vi "GetEdgeMenu.vi"(0 "reference":refnum<class "AbstractEdge.lvclass">, 5 "error in (no error)":errorcluster) -> (14 "reference out":refnum<class "AbstractEdge.lvclass">, 15 "MenuOptions":string[](array[string]), 19 "error out":errorcluster)   [LabVIEW 2014, in "AbstractEdge.lvclass"]
doc: "GetEdgeMenu"
uses:
  <resource>/Framework/Providers/Open_GDS/UML/AbstractEdge_class/AbstractEdge.lvclass
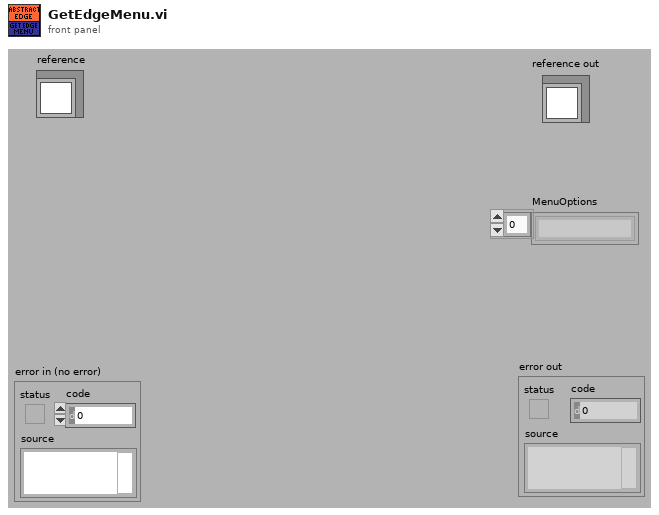
[diagram p1: front panel]
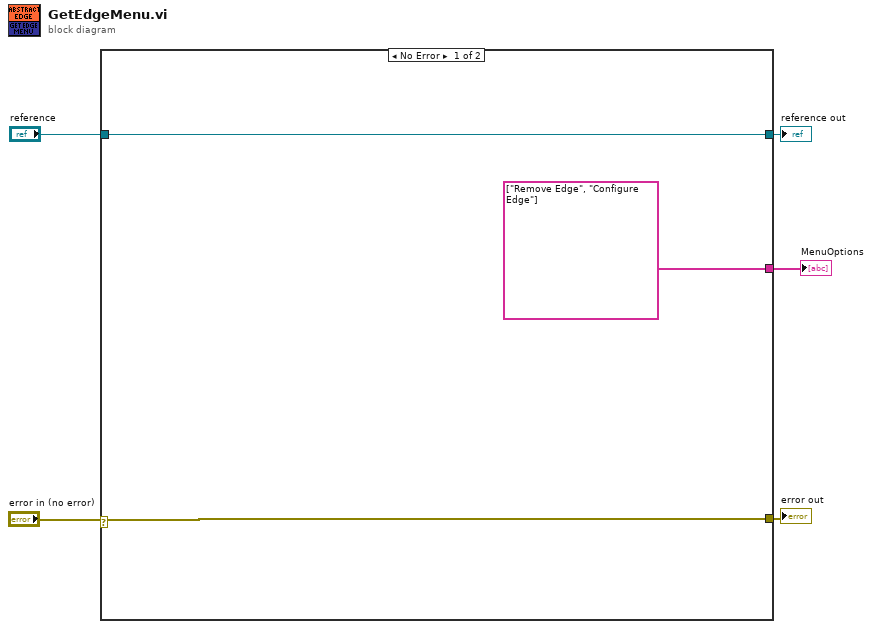
[diagram p0: block diagram]
diagram:
  n1 = case shown="No Error" "error in (no error)" {
    selector: "error in (no error)" -> [w7 w9]
    tunnel: "reference" -> [w8 w10]
    tunnel: [w7 w9] -> w4
    tunnel: [w8 w10] -> w3
    tunnel: [string[] ["Remove Edge", "Configure Edge"] _] -> w1
    frame No Error {
    }
    frame Error {
    }
  }
  "reference out" <- w3
  "error out" <- w4
  "MenuOptions" <- w1
